vi "List Resources.vi"(8 "error in (no error)":errorcluster, 11 "RP2040Target in":refnum<class "RP2040Target.lvclass">) -> (0 "error out":errorcluster, 2 "Resources":refnum<class "DeployResource.lvclass">[](array[class]), 3 "RP2040Target out":refnum<class "RP2040Target.lvclass">)   [LabVIEW 2020, in "RP2040.lvlib" / "RP2040Target.lvclass"]
uses:
  RP2040Target.lvclass
  Builds/picoG/ppl/PicoG-Core.lvlibp/DeployResource/DeployResource.lvclass
  VisaResource/VisaResource.lvclass
  C:/dev/Vireo/PicoG/Builds/picoG/ppl/PicoG-Core.lvlibp/DeployResource/DeployResource.lvclass
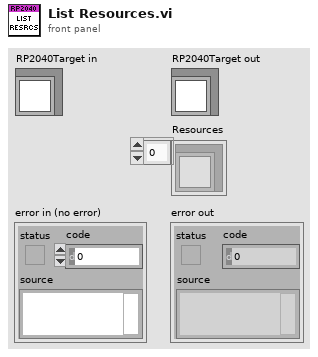
[diagram p1: front panel]
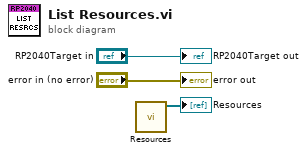
[diagram p0: block diagram]
diagram:
  n1 = call "Resources.vi"() -> ("Resources"=→"Resources":refnum<class "VisaResource.lvclass">[])  [unwired: 11 in]
  "error out" <- "error in (no error)"
  "RP2040Target out" <- "RP2040Target in"
